vi "Class.SaveCtrls.Restore.vi"(8 "error in":errorcluster, 11 "Save Control States in":refnum<class "Class.SaveCtrls.lvclass">) -> (0 "error out":errorcluster, 3 "Save Control States out":refnum<class "Class.SaveCtrls.lvclass">)   [LabVIEW 2024, in "EQMF.lvlib" / "Config Utils.lvlib" / "Class.SaveCtrls.lvclass"]
uses:
  Class.SaveCtrls.lvclass
  Class.SaveCtrls.lvclass/Class.SaveCtrls.ctl
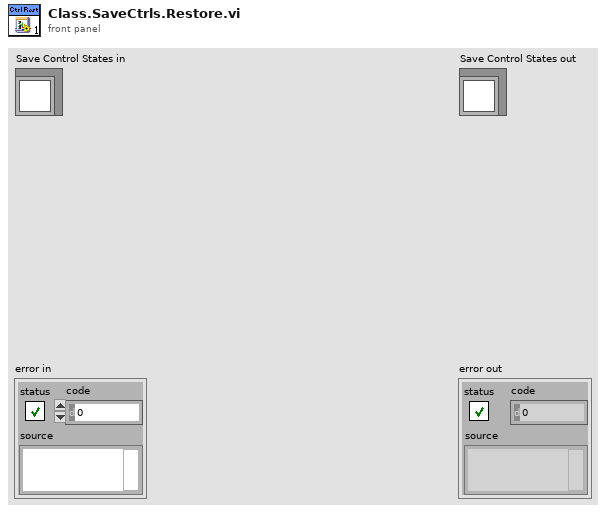
[diagram p1: front panel]
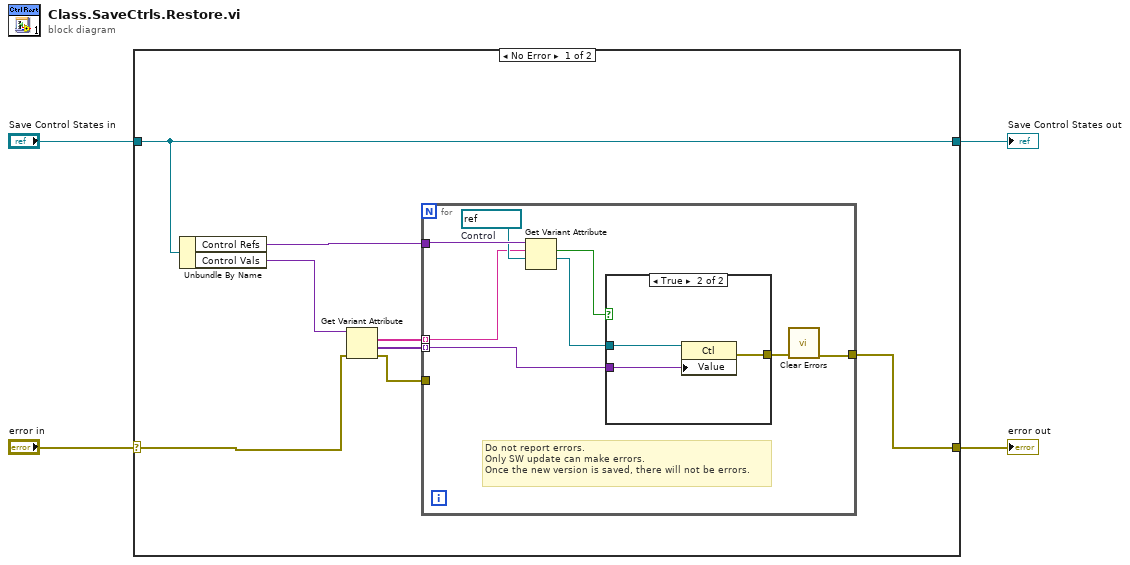
[diagram p0: block diagram]
diagram:
  n1 = case shown="No Error" "error in" {
    selector: "error in" -> [w8 w25]
    tunnel: [w7 w25] -> w3
    tunnel: [w12 w24] -> w1
    tunnel: "Save Control States in" -> [w12 w24]
    frame No Error {
      n2 = Unbundle By Name(w12) -> ("Control Refs"=w6:variant, "Control Vals"=w5:variant)
      n3 = Get Variant Attribute(Variant=w5, error in=w8) -> (names=w9:string[], values=w11:variant[], error out=w10:errorcluster)  [unwired: 2 in, 1 out]
      n4 = for {
        tunnel: w11 -> [w19] mode=indexing
        tunnel: w10 -> [_]
        tunnel: [w13] -> w7
        tunnel: w9 -> [w15] mode=indexing
        tunnel: w6 -> [w20]
        w18 = refnum<vi> refnum  # Control
        # "Do not report errors. \nOnly SW update can make errors.\nOnce the new version is saved, there will not be errors."
        n5 = Get Variant Attribute(Variant=w20, name=w15, default value (empty Variant)=w18) -> (found=w16:bool, value=w17:refnum<vi>)  [unwired: 1 in, 2 out]
        n6 = case shown="True" w16 {
          tunnel: [_ w23] -> w14
          tunnel: w19 -> [_ w22]
          tunnel: w17 -> [_ w21]
          frame False {
          }
          frame True {
            n7 = property class="Ctl"(reference=w21, "Value"=w22) -> (error out=w23:errorcluster)  [unwired: 1 in, 1 out]
          }
        }
        n8 = call <vilib>:"Clear Errors.vi"("error in (no error)"=w14) -> ("error out"=w13:errorcluster)  [unwired: 5 in, 1 out]
      }
    }
    frame Error {
    }
  }
  "error out" <- w3
  "Save Control States out" <- w1
